vi "Material-HelpDialog-Loadsheet.vi"() -> ()   [LabVIEW 2013, in "Material-RunTest.lvclass"]
uses:
  Material-RunTest.lvclass
panel:
  in  "OK Button":bool
  out "String":string="Pressing the Continue button will continue on with the same test with the same lot number. \n\nOn the last sheet in the LOT please press the last sheet in lot number button. \n\nAfter the last sheet in lot number button is pressed you will run the final sheet and then you will have to press begin test to test another Lot. \n\nIf you would like to cancel the test please press the cancel test button and the program will start from scratch. Press the begin button again to start testing."
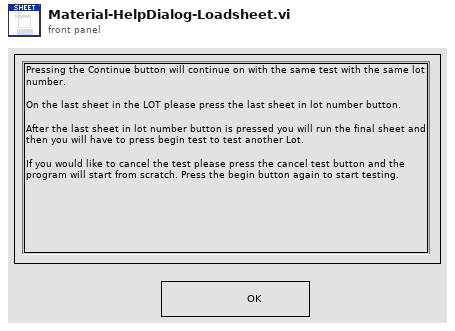
[diagram p1: front panel]
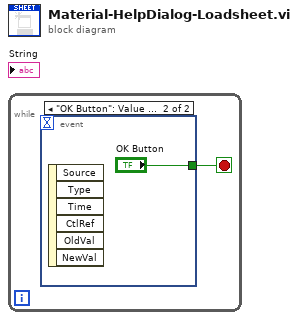
[diagram p0: block diagram]
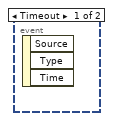
[diagram p2: hidden frame]
diagram:
  n1 = while {
    stop <- w1 stop-if-true
    n2 = event shown="[1] \"OK Button\": Value Change" {
      selector: _ -> [_ _]
      dyn-events: _ -> [_ _]
      timeout: _ -> [_ _]
      tunnel: [_ "OK Button"] -> w1
      event Timeout {
        n3 = event-data() -> ()  [unwired: 1 in, 3 out]
      }
      event "OK Button": Value Change {
        n4 = event-data() -> ()  [unwired: 1 in, 6 out]
      }
    }
  }
